vi "AprilTagCircle49h12IDList.vi"() -> (0 "Tag IDs":i32[](array[numeric]))   [LabVIEW 2020, in "g_ar_toolkit.feature_detection.lvlib"]
uses:
  g_ar_toolkit.feature_detection.lvlib
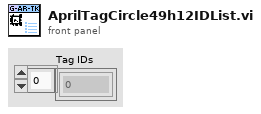
[diagram p1: front panel]
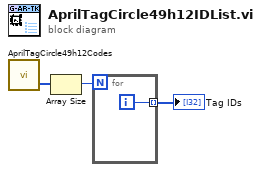
[diagram p0: block diagram]
diagram:
  n1 = call "AprilTagCircle49h12Codes.vi"() -> ("Codes"=w2:i64[])  [unwired: 2 in, 1 out]
  n2 = Array Size(array=w2) -> (size(s)=w3:i32)
  n3 = for {
    N: w3 -> [_]
    tunnel: [w4] -> w1 mode=indexing
    i -> [w4]
  }
  "Tag IDs" <- w1
